vi "AppConfig.vi"(8 "error in (no error)":errorcluster, 11 "ModelValidation":refnum<class "ModelValidationPlugin.lvclass">) -> (0 "error out":errorcluster, 3 "ModelValidation out":refnum<class "ModelValidationPlugin.lvclass">)   [LabVIEW 2017, in "AppPlugins.lvlib" / "ModelValidationPlugin.lvclass"]
uses:
  ModelValidationPlugin.lvclass
  ModelValidationPlugin.lvclass/ModelValidationPlugin.ctl
  Accessors/Read ModelValidationConfig.vi
  Accessors/Write ModelValidationConfig.vi
panel:
  in  "Initial condition":cluster{"H0":dbl, "xd0":dbl, "D0":dbl}={"H0"=4.55, "xd0"=0.275, "D0"=4.2}
  in  "Interpolation\n     Factor":i32=5
  in  "Offset Start \n     Time":dbl=2.0
  in  "Cancel Button":bool
  in  "Save Button":bool
  in  "Measurement\nNoiseVariance":dbl=0.001
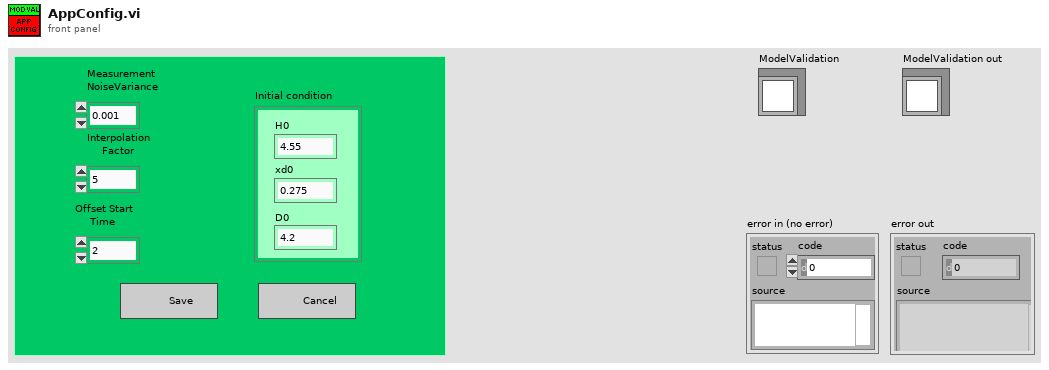
[diagram p1: front panel]
types:
  T1 = typedef "AppPlugins.lvlib/ModelValidationPlugin.lvclass/Config.ctl" = cluster{"NoiseVariance":dbl, "Iindex":i32, "OffsetTime":dbl, "InterpolationFactor":i32, "Initial condition":cluster{"H0":dbl, "xd0":dbl, "D0":dbl}}
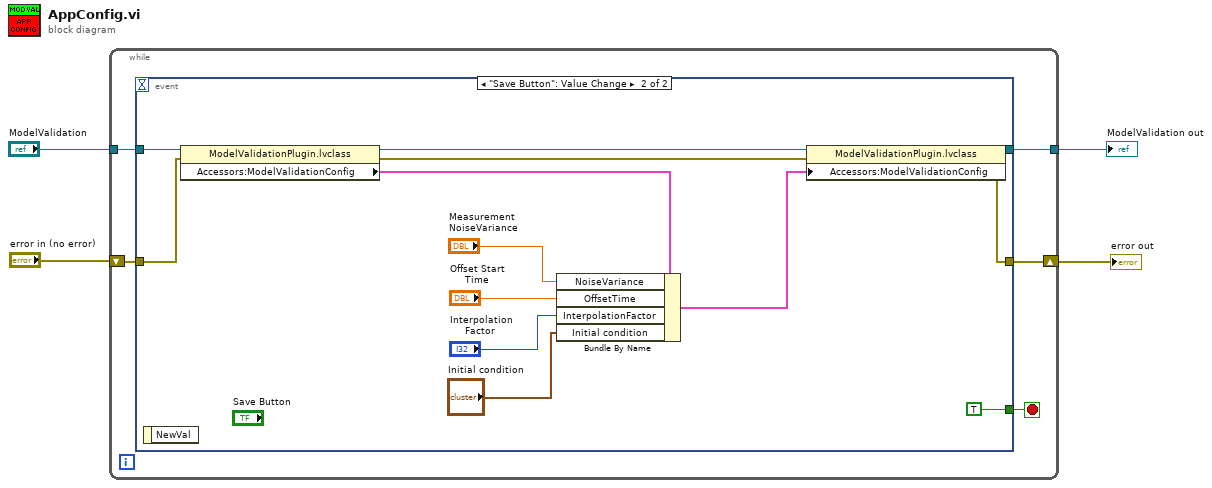
[diagram p0: block diagram]
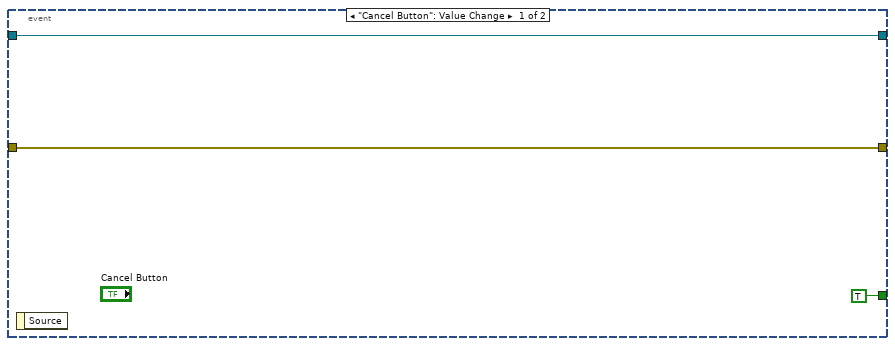
[diagram p2: hidden frame]
diagram:
  n1 = while {
    shift-right: [w9] -> w3
    shift-left: "error in (no error)" -> [w7]
    tunnel: [w8] -> w4
    tunnel: "ModelValidation" -> [w5]
    stop <- w6 stop-if-true
    n2 = event shown="[1] \"Save Button\": Value Change" {
      selector: _ -> [_ _]
      dyn-events: _ -> [_ _]
      timeout: _ -> [_ _]
      tunnel: [w12 w25] -> w9
      tunnel: [w10 w24] -> w8
      tunnel: w7 -> [w12 w21]
      tunnel: [TRUE TRUE] -> w6
      tunnel: w5 -> [w10 w17]
      event "Cancel Button": Value Change {
        n3 = event-data() -> ()  [unwired: 1 in, 1 out]
      }
      event "Save Button": Value Change {
        n4 = event-data() -> ()  [unwired: 1 in, 1 out]
        n5 = property class="ModelValidationPlugin.lvclass"(reference=w17, error in=w21) -> (reference out=w22:refnum<class "ModelValidationPlugin.lvclass">, error out=w20:errorcluster, "Accessors:ModelValidationConfig"=w19:T1)
        n6 = Bundle By Name(cluster=w19, "NoiseVariance"="Measurement\nNoiseVariance", "OffsetTime"="Offset Start \n     Time", "InterpolationFactor"="Interpolation\n     Factor", "Initial condition"="Initial condition") -> (w18:T1)
        n7 = property class="ModelValidationPlugin.lvclass"(reference=w22, error in=w20, "Accessors:ModelValidationConfig"=w18) -> (reference out=w24:refnum<class "ModelValidationPlugin.lvclass">, error out=w25:errorcluster)
      }
    }
  }
  "error out" <- w3
  "ModelValidation out" <- w4
